vi "Dashboard Main.vi"() -> ()   [LabVIEW 2012]
uses:
  Auto State Selector.ctl
  Level state.ctl
  <vilib>/Utility/config.llb/Read Key (String).vi
  <vilib>/Utility/config.llb/Read Key (I32).vi
  <vilib>/Utility/config.llb/Write Key (String).vi
  <vilib>/Utility/config.llb/Write Key (I32).vi
  <vilib>/Utility/config.llb/NI_LVConfig.lvlib
panel:
  out "Dumping":bool
  out "Side Ramp":bool
  out "Pawl Extended":bool
  out "Small Hooks Extended":bool
  in  "Level Selector":T1
  out "Bail Climb":bool
  out "Big Hooks on Bar":bool
  in  "Auto State Selector":T2
  out "Climbing":bool
  in  "Camera Settings":T3={"Frate Rate"=30, "Compression"=30, "Size"=1} {"Frate Rate" scale=1.0..30.0; "Size" items=["640x480", "320x240", "160x120"]}
  out "Mode":T4(ring)=enum."Auto Disabled"
  out "Camera IP":string
  in  "Viewer":enum32{"Camera Image"}(tab)
  out "Mbps":dbl format="%#.1g"
  in  "Enable":bool
  in  "DB Camera Config":bool
  out "Mbps":bool
  out "fps":dbl format="%#.1g"
  out "Image Error Message":string="Timeout in Camera Communications"
  out "Camera Image":T5(plugin-control)
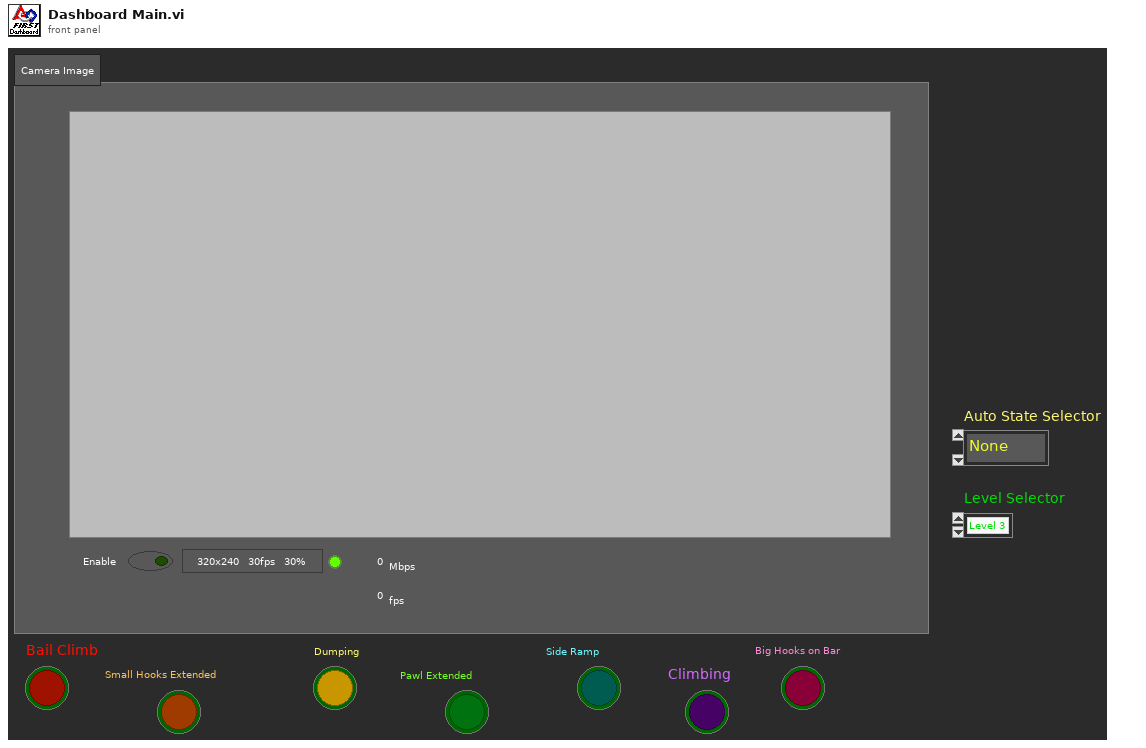
[diagram p1: front panel]
types:
  T1 = typedef "Level state.ctl" = enum16{"Level 3", "Level 2", "Level 1"}
  T2 = typedef "Auto State Selector.ctl" = enum16{"None", "Fire 2x", "Fire 3x", "Dump in low goal"}
  T3 = cluster{"Frate Rate":i32, "Compression":i32, "Size":u16}
  T4 = enum8{"Tele-Op Disabled", "Tele-Op Enabled", "Auto Disabled", "Auto Enabled", "Test Disabled", "Test Enabled", ""}
  T5 = typedef "IMAQ Image.ctl" = refnum<image>
  T6 = typedef "Image Type" = u32
  T7 = typedef "LVRectTypeDef.ctl" = cluster{"Left":i16, "Top":i16, "Right":i16, "Bottom":i16}
  T8 = cluster{"Competition mode":bool, "Robot Link":bool, "Autonomous":bool, "Enabled":bool, "E-Stop":bool, "Simulated":bool, "TestMode":bool, "Docked Window":bool}
  T9 = typedef "NI_LVConfig.lvlib/Config Data RefNum.ctl" = refnum<k1>
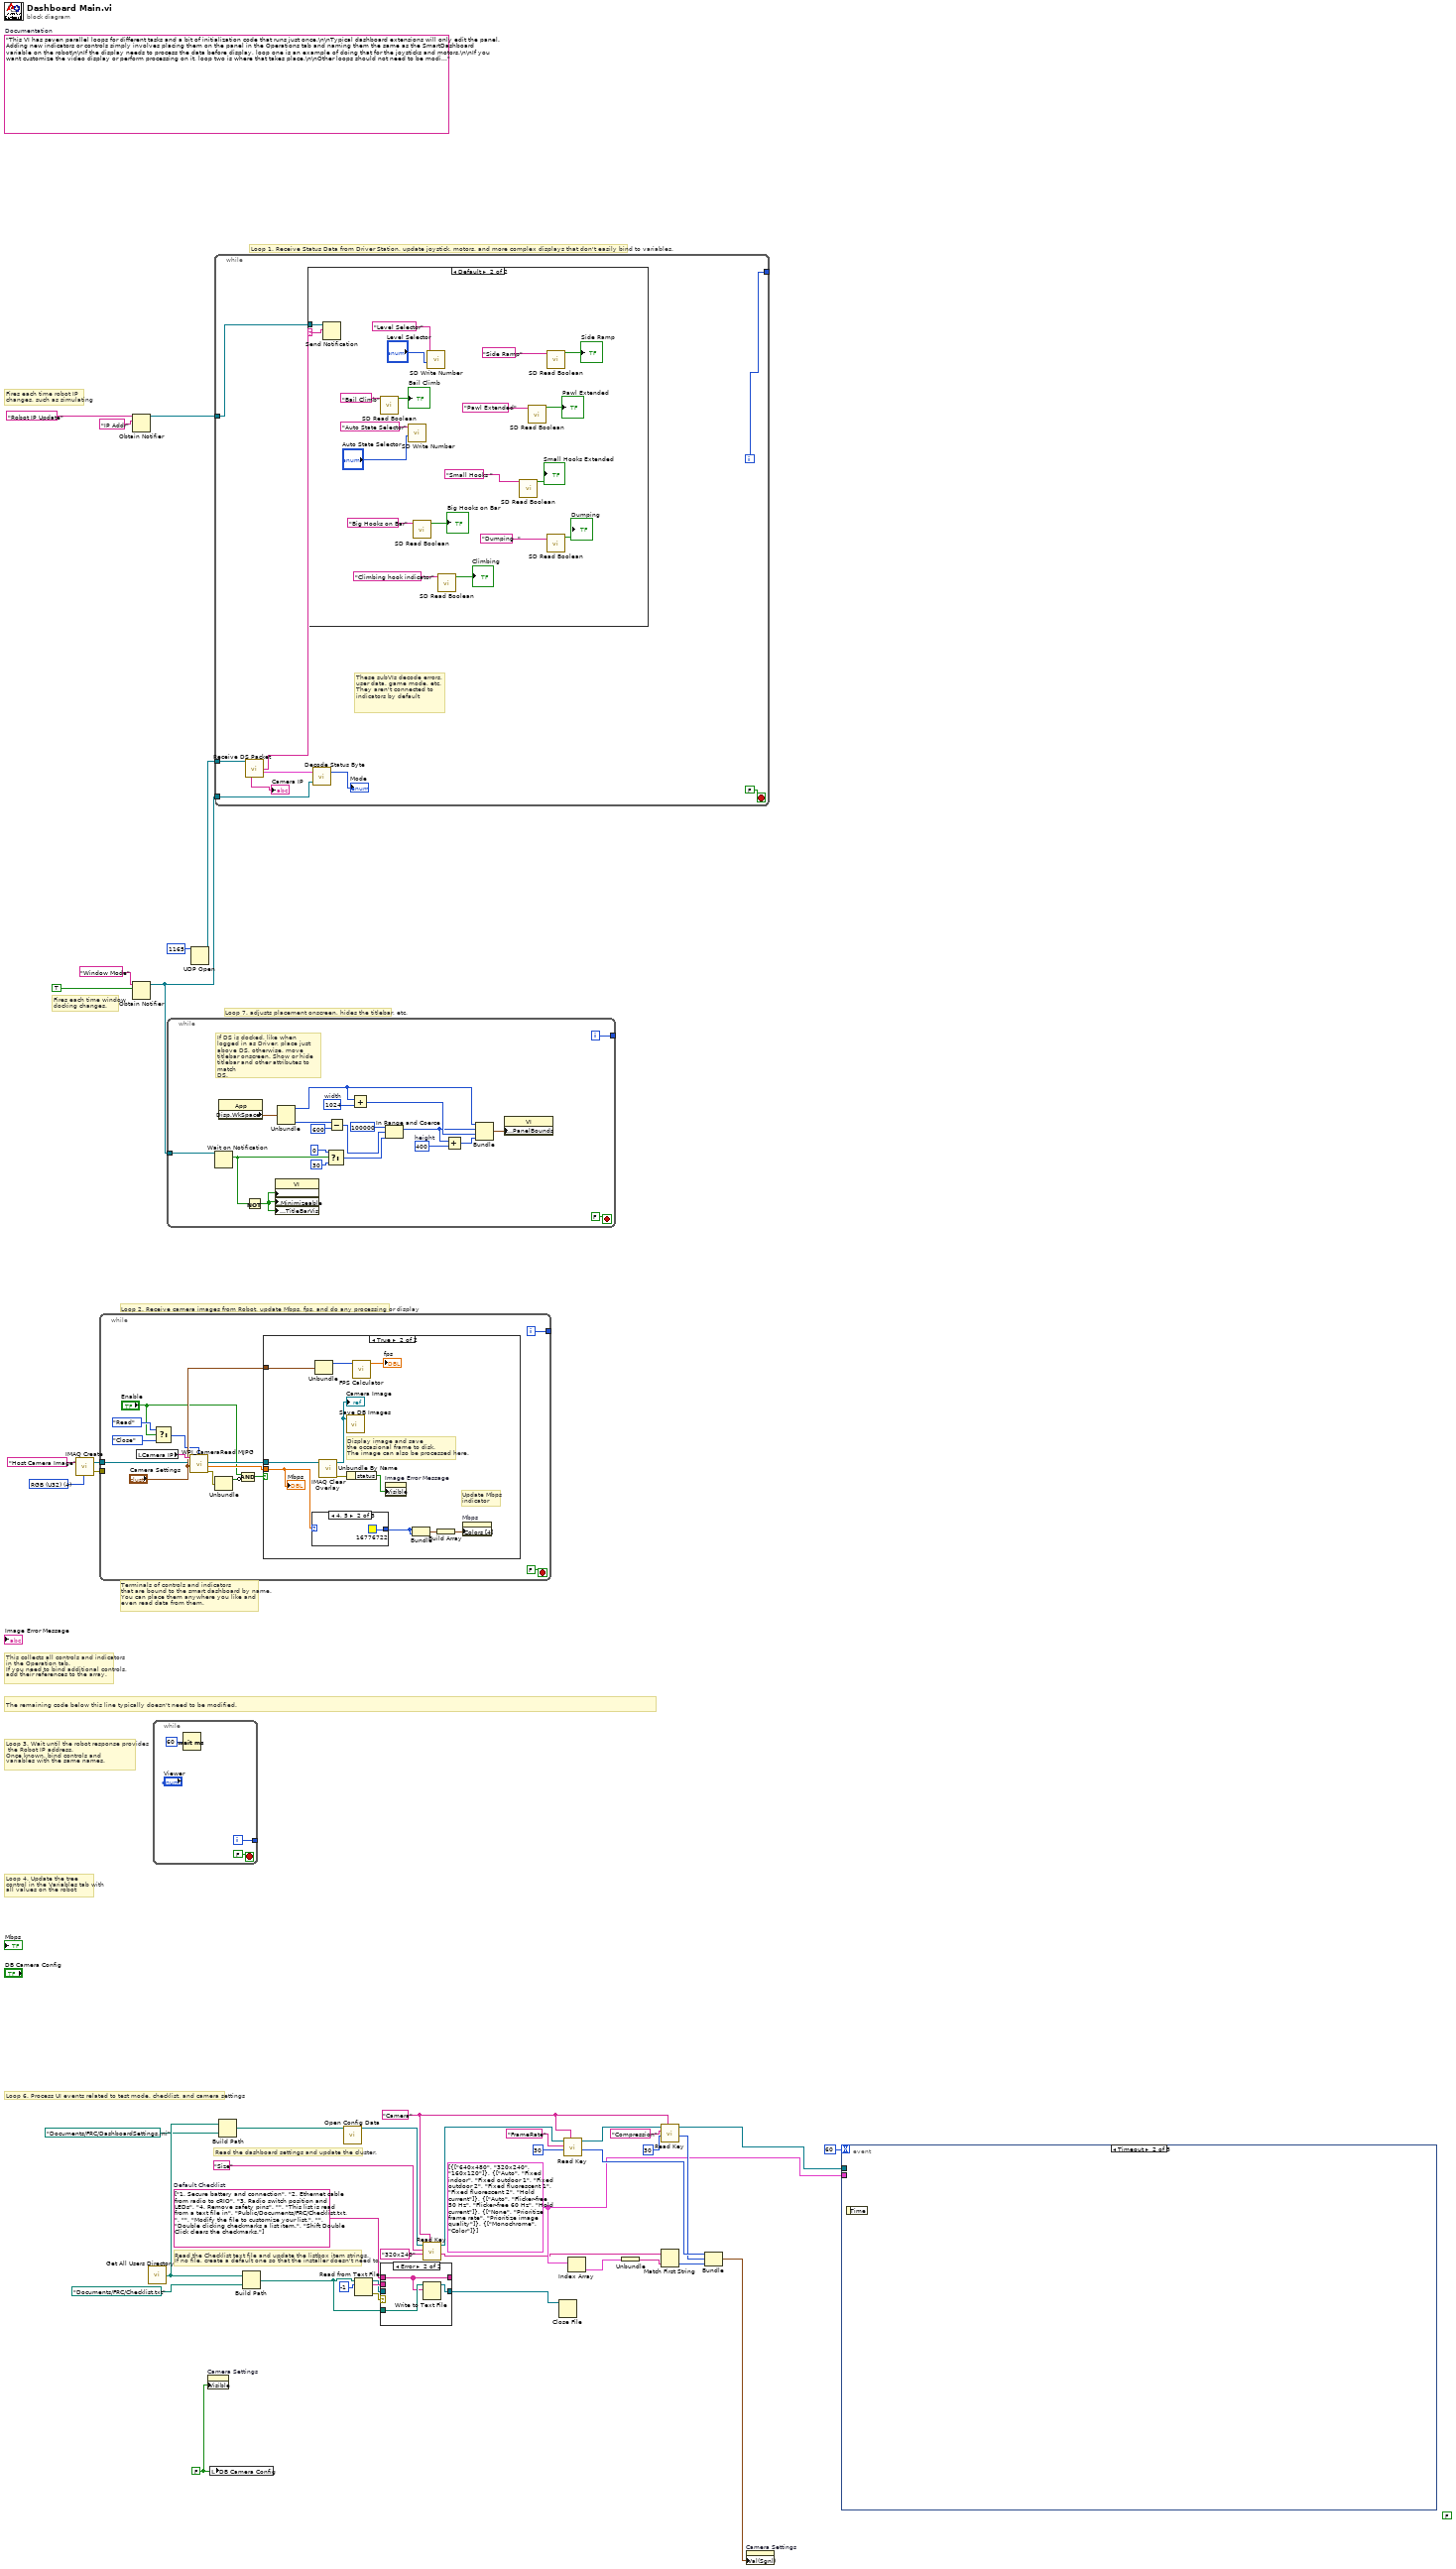
[diagram p0: block diagram]
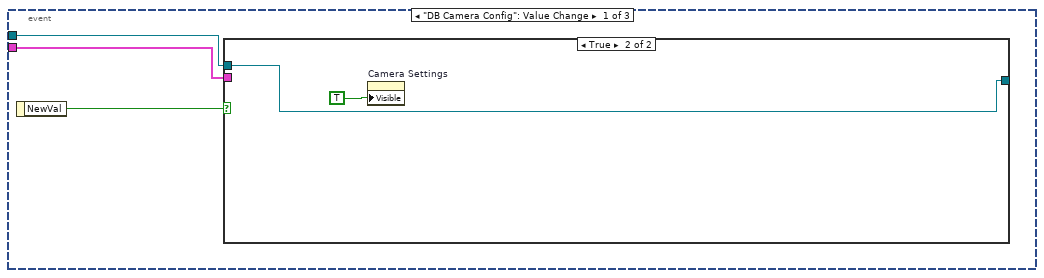
[diagram p2: hidden frame]
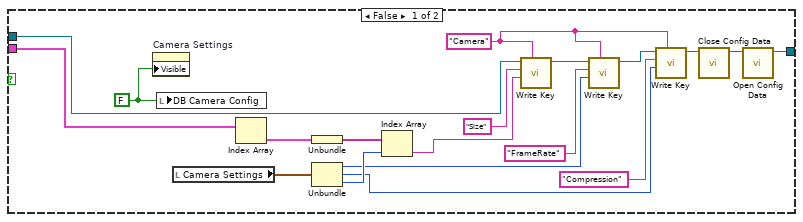
[diagram p3: hidden frame]
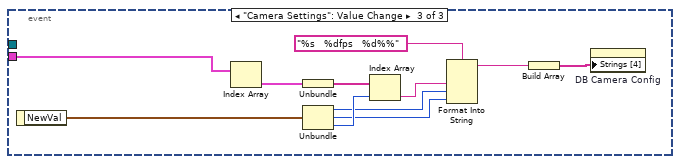
[diagram p4: hidden frame]
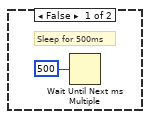
[diagram p5: hidden frame]
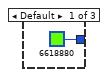
[diagram p6: hidden frame]
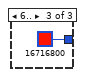
[diagram p7: hidden frame]
diagram:
  (unwired) FALSE
  w21 = "Camera"
  w13 = cluster{string[]}[] [{["640x480", "320x240", "160x120"]}, {["Auto", "Fixed indoor", "Fixed outdoor 1", "Fixed outdoor 2", "Fixed fluorescent 1", "Fixed fluorescent 2", "Hold current"]}, {["Auto", "Flicker-free 50 Hz", "Flicker-free 60 Hz", "Hold current"]}, {["None", "Prioritize frame rate", "Prioritize image quality"]}, {["Monochrome", "Color"]}]
  w28 = string[] ["1. Secure battery and connection", "2. Ethernet cable from radio to cRIO", "3. Radio switch position and LEDs", "4. Remove safety pins", "", "This list is read from a text file in", "Public/Documents/FRC/Checklist.txt.", "", "Modify the file to customize your list.", "", "Double clicking checkmarks a list item.", "Shift Double Click clears the checkmarks."]  # Default Checklist
  w27 = FALSE ("Visible")
  (unwired) "This VI has seven parallel loops for different tasks and a bit of initialization code that runs just once.\n\nTypical dashboard extensions will only edit the panel. Adding new indicators or controls simply involves placing them on the panel in the Operations tab and naming them the same as the SmartDashboard variable on the robot\n\nIf the display needs to process the data before display, loop one is an example of doing that for the joysticks and motors.\n\nIf you want customize the video display or perform processing on it, loop two is where that takes place.\n\nOther loops should not need to be modified. They are pretty standard, and document the task they perform."  # Documentation
  w42 = T6 4 items=["Grayscale (U8)", "Grayscale (I16)", "Grayscale (SGL)", "Complex (CSG)", "RGB (U32)", "HSL (U32)", "RGB (U64)"] ("Image Type")
  # "Fires each time robot IP\nchanges, such as simulating"
  # "Fires each time window\ndocking changes."
  # "Read the Checklist text file and update the listbox item strings.\nIf no file, create a default one so that the installer doesn't need to."
  # "This collects all controls and indicators\nin the Operation tab.\nIf you need to bind additional controls,\nadd their references to the array."
  # "The remaining code below this line typically doesn't need to be modified."
  # "Loop 6. Process UI events related to test mode, checklist, and camera settings"
  # "Read the dashboard settings and update the cluster."
  # "Terminals of controls and indicators\nthat are bound to the smart dashboard by name.\nYou can place them anywhere you like and\neven read data from them."
  # "Loop 4. Update the tree\ncontrol in the Variables tab with\nall values on the robot"
  # "Loop 3. Wait until the robot response provides\n the Robot IP address.\nOnce known, bind controls and\nvariables with the same names."
  # "Loop 7. adjusts placement onscreen, hides the titlebar, etc."
  # "Loop 1. Receive Status Data from Driver Station, update joystick, motors, and more complex displays that don't easily bind to variables."
  # "Loop 2. Receive camera images from Robot, update Mbps, fps, and do any processing or display"
  n1 = call "IMAQ Create"("Image Name"="Host Camera Image", "Image Type"=w42) -> ("New Image"=w40:T5, "error out"=w39:errorcluster)  [unwired: 2 in, 1 out]
  n2 = while {
    tunnel: w40 -> [w54]
    tunnel: w39 -> [_]
    tunnel: [w57] -> _
    i -> [w57]
    stop <- FALSE stop-if-true
    n3 = local read "Camera IP"() -> (w56:string)
    n4 = Select(t=enum16{"Read", "Reopen", "Close"}."Read" ("Operation"), s="Enable", f=enum16{"Read", "Reopen", "Close"}."Close" ("Operation")) -> (s? t:f=w49:enum16{"Read", "Reopen", "Close"})
    n5 = call <vilib>:"WPI_CameraRead MJPG.vi"("Operation"=w49, "Camera Settings"="Camera Settings", "Image"=w54, "address"=w56) -> ("error out"=w48:errorcluster, "Bandwidth (kbps)"=w52:dbl, "Image Out"=w53:T5)  [unwired: 5 in]
    n6 = Unbundle(w48) -> ("status"=w46:bool)  [unwired: 2 out]
    n7 = Compound Arithmetic op=AND("Enable", invert w46) -> (w45:bool)
    n8 = case shown="True" w45 {
      tunnel: "Camera Settings" -> [_ w61]
      tunnel: w53 -> [_ w64]
      tunnel: w52 -> [_ w63]
      frame False {
        # "Sleep for 500ms"
        n9 = Wait Until Next ms Multiple(millisecond multiple=u32 500) -> ()  [unwired: 1 out]
      }
      frame True {
        # "Display image and save\nthe occasional frame to disk.\nThe image can also be processed here."
        # "Update Mbps\nindicator"
        n10 = case shown="4, 5" w63 {
          tunnel: [u32 6618880 ("Color Box") u32 16776722 ("Color Box") u32 16716800 ("Color Box")] -> w65
          frame Default {
          }
          frame 4, 5 {
          }
          frame 6.. {
          }
        }
        n11 = Unbundle(w61) -> ("Frate Rate"=w60:i32)  [unwired: 2 out]
        n12 = call "IMAQ Clear Overlay"("Image"=w64) -> ("error out"=w69:errorcluster, "Image Out"=w68:T5)  [unwired: 2 in, 7 out]
        "Camera Image" <- w68
        n13 = call "Save DB Images.vi"("Image"=w68) -> ()  [unwired: 2 in, 1 out]
        n14 = Unbundle By Name(w69) -> ("status"=w70:bool)
        n15 = call "FPS Calculator.vi"("Average Count"=w60) -> ("fps"=→"fps":dbl)  [unwired: 10 in]
        n16 = property on="Image Error Message" class="Str"("Visible"=w70) -> ()  [unwired: 2 in, 2 out]
        n17 = Bundle("Color Box"=w65, "Color Box"=w65) -> (w67:cluster{"Color Box":u32, "Color Box":u32})  [unwired: 1 out]
        n18 = Build Array(w67) -> (w66:cluster{"Color Box":u32, "Color Box":u32}[])
        n19 = property on="Mbps" class="Bool (strict)"("Colors [4]"=w66) -> ()  [unwired: 2 in, 2 out]
        "Mbps" <- w63
      }
    }
  }
  n20 = Obtain Notifier(name (unnamed)="Robot IP Update", notification data type="IP Addr" ("name (unnamed)")) -> (notifier out=w1:refnum<notifier>)  [unwired: 2 in, 2 out]
  n21 = Obtain Notifier(name (unnamed)="Window Mode", notification data type=TRUE) -> (notifier out=w32:refnum<notifier>)  [unwired: 2 in, 2 out]
  n22 = call "Get All Users Directory.vi"() -> ("All User Path"=w26:path)
  n23 = while {
    tunnel: [w74] -> _
    i -> [w74]
    stop <- FALSE stop-if-true
    n24 = Wait (ms)(milliseconds to wait=u32 60) -> ()  [unwired: 1 out]
  }
  n25 = while {
    tunnel: w32 -> [w95]
    tunnel: [w93] -> _
    i -> [w93]
    stop <- FALSE stop-if-true
    w85 = 1024  # width
    w88 = 400  # height
    # "If DS is docked, like when\nlogged in as Driver, place just\nabove DS, otherwise, move\ntitlebar onscreen. Show or hide\ntitlebar and other attributes to match\nDS."
    n26 = Wait on Notification(notifier=w95) -> (notification=w80:bool)  [unwired: 3 in, 3 out]
    n27 = property class="App"() -> ("Disp.WkSpace"=w91:T7)  [unwired: 2 in, 2 out]
    n28 = Not(x=w80) -> (.not. x?=w94:bool)
    n29 = property class="VI"("Front Panel.Closeable"=w94, "Front Panel.Minimizeable"=w94, "Front Panel.TitleBarVis"=w94) -> ()  [unwired: 2 in, 2 out]
    n30 = Unbundle(w91) -> ("Left"=w89:i16, "Bottom"=w86:i16)  [unwired: 2 out]
    n31 = Select(t=0, s=w80, f=30) -> (s? t:f=w79:i32)
    n32 = Subtract(x=w86, y=600) -> (x-y=w83:i32)
    n33 = Add(x=w89, y=w85) -> (x+y=w90:i32)
    n34 = In Range and Coerce(upper limit=100000, x=w83, lower limit=w79) -> (coerced(x)=w77:i32)  [unwired: 1 out]
    n35 = Add(x=w77, y=w88) -> (x+y=w87:i32)
    n36 = Bundle("Left"=w89, w77, w90, w87) -> (w92:cluster{"Left":i16, i32, i32, i32})  [unwired: 1 out]
    n37 = property class="VI"("Front Panel.PanelBounds"=w92) -> ()  [unwired: 2 in, 2 out]
  }
  n38 = UDP Open(11:u16 1165 ("port")) -> (port=w43:refnum<k16>)  [unwired: 2 in, 4 out]
  n39 = property on="Camera Settings" class="Clust (strict)"("Visible"=w27) -> ()  [unwired: 2 in, 2 out]
  n40 = local write "DB Camera Config"(w27) -> ()
  n41 = while {
    tunnel: w43 -> [w103]
    tunnel: w1 -> [w98]
    tunnel: w32 -> [w102]
    tunnel: [w99] -> _
    i -> [w99]
    stop <- FALSE stop-if-true
    # "These subVIs decode errors, user data, game mode, etc.\nThey aren't connected to indicators by default"
    n42 = call "Receive DS Packet.vi"("Recv Socket"=w103) -> ("Robot IP Address"=w97:string, "Status"=w104:T8, "Camera IP Address"=→"Camera IP":string)  [unwired: 1 in, 11 out]
    n43 = case shown="Default" w97 {
      selector: w97 -> [_ w124]
      tunnel: w98 -> [_ w125]
      frame "0.0.0.0" {
        # "Robot not responding, don't poll the variables"
      }
      frame Default {
        n44 = Send Notification(notification=w124, notifier=w125) -> ()  [unwired: 1 in, 2 out]
        n45 = call <vilib>:"SD Read Boolean.vi"("Name"="Bail Climb") -> ("Boolean"=→"Bail Climb":bool)  [unwired: 8 in, 2 out]
        n46 = call <vilib>:"SD Write Number.vi"("Numeric"="Auto State Selector", "Name"="Auto State Selector") -> ()  [unwired: 8 in, 2 out]
        n47 = call <vilib>:"SD Read Boolean.vi"("Name"="Big Hooks on Bar") -> ("Boolean"=→"Big Hooks on Bar":bool)  [unwired: 8 in, 2 out]
        n48 = call <vilib>:"SD Write Number.vi"("Numeric"="Level Selector", "Name"="Level Selector") -> ()  [unwired: 8 in, 2 out]
        n49 = call <vilib>:"SD Read Boolean.vi"("Name"="Climbing hook indicator") -> ("Boolean"=→"Climbing":bool)  [unwired: 8 in, 2 out]
        n50 = call <vilib>:"SD Read Boolean.vi"("Name"="Small Hooks ") -> ("Boolean"=→"Small Hooks Extended":bool)  [unwired: 8 in, 2 out]
        n51 = call <vilib>:"SD Read Boolean.vi"("Name"="Pawl Extended") -> ("Boolean"=→"Pawl Extended":bool)  [unwired: 8 in, 2 out]
        n52 = call <vilib>:"SD Read Boolean.vi"("Name"="Side Ramp") -> ("Boolean"=→"Side Ramp":bool)  [unwired: 8 in, 2 out]
        n53 = call <vilib>:"SD Read Boolean.vi"("Name"="Dumping  ") -> ("Boolean"=→"Dumping":bool)  [unwired: 8 in, 2 out]
      }
    }
    n54 = call "Decode Status Byte.vi"("Window Mode Notifier"=w102, "Status"=w104) -> ("Mode"=→"Mode":T4)  [unwired: 1 out]
  }
  n55 = Build Path(base path=w26, name or relative path=path "Documents/FRC/DashboardSettings.ini") -> (appended path=w25:path)
  n56 = Build Path(base path=w26, name or relative path=path "Documents/FRC/Checklist.txt") -> (appended path=w29:path)
  n57 = call <vilib>:"Open Config Data.vi"("configuration file path"=w25) -> ("refnum"=w24:T9)  [unwired: 8 in, 2 out]
  n58 = Read from Text File(file (use dialog)=w29, count=-1 ("timeout ms (25000)")) -> (refnum out=w8:refnum<file>, text=w30:string[], error out=w31:errorcluster)  [unwired: 2 in, 1 out]
  n59 = case shown="Error" w31 {
    tunnel: w30 -> [w127 _]
    tunnel: [w127 w129] -> _
    tunnel: w28 -> [_ w129]
    tunnel: w29 -> [_ w130]
    tunnel: [w126 w128] -> w7
    tunnel: w8 -> [w126 _]
    frame No Error {
    }
    frame Error {
      n60 = Write to Text File(file (use dialog)=w130, text=w129) -> (refnum out=w128:refnum<file>)  [unwired: 2 in, 2 out]
    }
  }
  n61 = call-poly <vilib>:"Read Key.vi"("section"=w21, "default value"="320x240", "key"="Size", "refnum"=w24) -> ("value"=w11:string, "refnum out"=w6:T9)  [unwired: 2 in, 4 out]
  n62 = Close File(refnum=w7) -> ()  [unwired: 1 in, 2 out]
  n63 = call-poly <vilib>:"Read Key.vi"("section"=w21, "default value"=30, "key"="FrameRate", "refnum"=w6) -> ("value"=w16:i32, "refnum out"=w5:T9)  [unwired: 1 in, 5 out]
  n64 = Index Array(array=w13) -> (element=w14:cluster{string[]})  [unwired: 1 in]
  n65 = Unbundle(w14) -> (w12:string[])
  n66 = call-poly <vilib>:"Read Key.vi"("section"=w21, "default value"=30, "key"="Compression", "refnum"=w5) -> ("value"=w15:i32, "refnum out"=w3:T9)  [unwired: 1 in, 5 out]
  n67 = Match First String(2:w12, 3:w11) -> (0:w10:i32)  [unwired: 1 out]
  n68 = Bundle("value"=w16, "value"=w15, "index"=w10) -> (w4:cluster{"value":i32, "value":i32, "index":i32})  [unwired: 1 out]
  n69 = property on="Camera Settings" class="Clust (strict)"("Val(Sgnl)"=w4) -> ()  [unwired: 2 in, 2 out]
  n70 = event shown="[1] Timeout" {
    selector: _ -> [_ _ _]
    dyn-events: _ -> [_ _ _]
    timeout: u32 60 ("milliseconds to wait") -> [_ _ _]
    tunnel: w13 -> [w132 _ w161]
    tunnel: w3 -> [w131 _ _]
    event "DB Camera Config": Value Change {
      n71 = event-data() -> ("NewVal"=w133:bool)  [unwired: 1 in]
      n72 = case shown="True" w133 {
        tunnel: w132 -> [w142 _]
        tunnel: [w135 w153] -> _
        tunnel: w131 -> [w134 w153]
        frame False {
          w149 = "Camera"
          w152 = FALSE ("Visible")
          n73 = property on="Camera Settings" class="Clust (strict)"("Visible"=w152) -> ()  [unwired: 2 in, 2 out]
          n74 = local write "DB Camera Config"(w152) -> ()
          n75 = local read "Camera Settings"() -> (w141:T3)
          n76 = Index Array(array=w142) -> (element=w145:cluster{string[]})  [unwired: 1 in]
          n77 = Unbundle(w145) -> (w144:string[])
          n78 = Unbundle(w141) -> ("Frate Rate"=w140:i32, "Compression"=w139:i32, "Size"=w143:u16)
          n79 = Index Array(array=w144, index=w143) -> (element=w138:string)
          n80 = call-poly <vilib>:"Write Key.vi"("section"=w149, "value"=w138, "key"="Size", "refnum"=w134) -> ("refnum out"=w151:T9)  [unwired: 2 in, 5 out]
          n81 = call-poly <vilib>:"Write Key.vi"("section"=w149, "value"=w140, "key"="FrameRate", "refnum"=w151) -> ("refnum out"=w150:T9)  [unwired: 1 in, 6 out]
          n82 = call-poly <vilib>:"Write Key.vi"("section"=w149, "value"=w139, "key"="Compression", "refnum"=w150) -> ("refnum out"=w136:T9)  [unwired: 1 in, 6 out]
          n83 = call <vilib>:"Close Config Data.vi"("refnum"=w136) -> ("file path"=w137:path)  [unwired: 2 in, 8 out]
          n84 = call <vilib>:"Open Config Data.vi"("configuration file path"=w137) -> ("refnum"=w135:T9)  [unwired: 8 in, 2 out]
        }
        frame True {
          n85 = property on="Camera Settings" class="Clust (strict)"("Visible"=TRUE) -> ()  [unwired: 2 in, 2 out]
        }
      }
    }
    event Timeout {
      n86 = event-data() -> ()  [unwired: 1 in, 1 out]
    }
    event "Camera Settings": Value Change {
      n87 = event-data() -> ("NewVal"=w165:T3)  [unwired: 1 in]
      n88 = Index Array(array=w161) -> (element=w160:cluster{string[]})  [unwired: 1 in]
      n89 = Unbundle(w160) -> (w159:string[])
      n90 = Unbundle(w165) -> ("Frate Rate"=w156:i32, "Compression"=w155:i32, "Size"=w158:u16)
      n91 = Index Array(array=w159, index=w158) -> (element=w157:string)
      n92 = Format Into String(format string="%s   %dfps   %d%%", w157, w156, w155) -> (resulting string=w162:string)  [unwired: 2 in, 1 out]
      n93 = Build Array(w162) -> (w163:string[])
      n94 = property on="DB Camera Config" class="Bool (strict)"("Strings [4]"=w163) -> ()  [unwired: 2 in, 2 out]
    }
  }
